vi "VdDigitalControl_Simulated_Create.vi"(8 "Error In":errorcluster, 10 "Address":string, 11 "reference in":refnum<class "VdDigitalControl_Simulated.lvclass">) -> (0 "Error Out":errorcluster, 3 "reference out":refnum<class "VdDigitalControl_Simulated.lvclass">)   [LabVIEW 2020, in "VdDigitalControl_Simulated.lvclass"]
uses:
  VdDigitalControl_Simulated.lvclass
  C:/Projects/OpenGDS_DesignPatterns/Factory1/VdDigitalControl_class/VdDigitalControl.lvclass
  VdDigitalControl_Simulated.lvclass/VdDigitalControl_Simulated.ctl
  VdDigitalControl_class/VdDigitalControl.lvclass
  C:/Projects/OpenGDS_DesignPatterns/Factory1/VdInstrument_class/VdInstrument.lvclass
  C:/Projects/OpenGDS_DesignPatterns/Factory1/VdDigitalControl_Simulated_class/VdDigitalControl_Simulated.lvclass
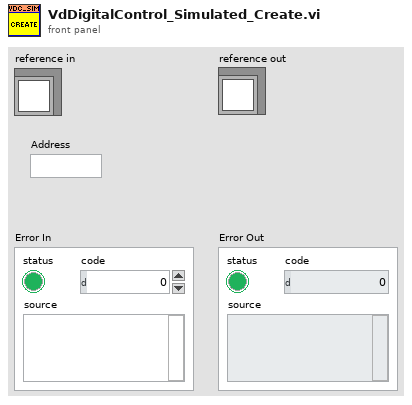
[diagram p1: front panel]
types:
  T1 = typedef "VdDigitalControl_Simulated.lvclass/ObjectAttributes.ctl" = cluster{"None":bool}
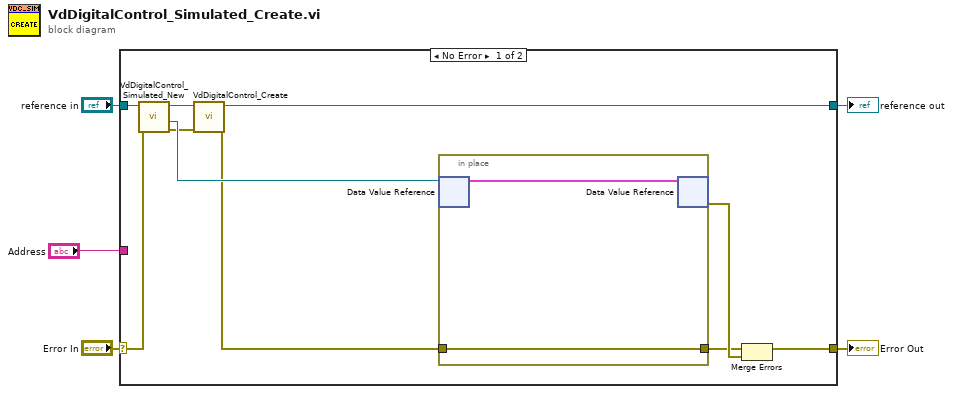
[diagram p0: block diagram]
diagram:
  n1 = case shown="No Error" "Error In" {
    selector: "Error In" -> [w11 w19]
    tunnel: [w9 w19] -> w4
    tunnel: "reference in" -> [w13 w18]
    tunnel: [w8 w18] -> w2
    tunnel: "Address" -> [_ _]
    frame No Error {
      n2 = call "VdDigitalControl_Simulated_New.vi"("error in (no error)"=w11, "reference in"=w13) -> ("error out"=w12:errorcluster, "DVRRefOut"=w15:refnum<data-value>, "reference out"=w14:refnum<class "VdDigitalControl_Simulated.lvclass">)  [unwired: 6 in, 1 out]
      n3 = call "VdDigitalControl_Create.vi"("Error In"=w12, "reference in"=w14) -> ("Error Out"=w6:errorcluster, "reference out"=w8:refnum<class "VdDigitalControl_Simulated.lvclass">)  [unwired: 8 in]
      n4 = in-place {
        in-place-border: w6 -> [w17]
        in-place-border: [w17] -> w7
        n5 = in-place-dvr #1(w15) -> (w16:T1)  [unwired: 1 out]
        n6 = in-place-dvr #1(w16) -> (w10:errorcluster)  [unwired: 1 out]
      }
      n7 = Merge Errors(w7, w10) -> (w9:errorcluster)
    }
    frame Error {
    }
  }
  "Error Out" <- w4
  "reference out" <- w2
